vi "subSave_PatchParams_New.vi"(9 "Scaled output":cluster{"xo":i32, dbl, "data":dbl[][]}(graph)={"xo"=0, 5e-05, "data"=array2x40000[80000 elements]}, 10 "Patch quality":T1={"Ra (MΩ)"=236.79401827082728, "Rm (MΩ)"=5201.968657026799, "Cm (pF)"=4.323624616129607, "RC constant (msec)"=1.0238084463479926, "Steady state current (pA)"=9.611745724853648}, 11 "Base path":path=path "C:/Peng/Data/2014-05-13 neuron PZ066 DRH344/DRH344/fov2") -> ()   [LabVIEW 2015]
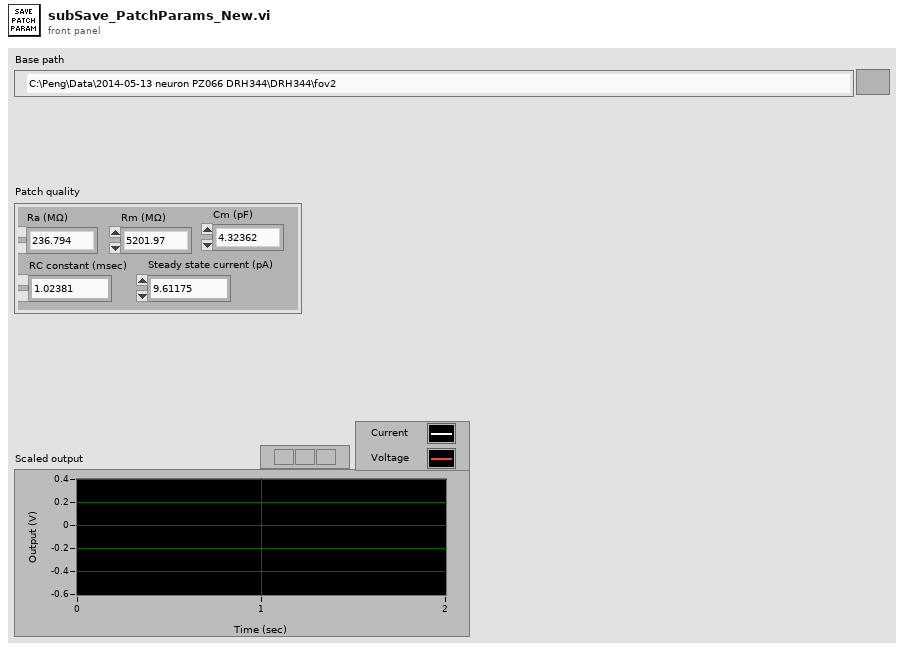
[diagram p1: front panel]
types:
  T1 = cluster{"Ra (MΩ)":dbl, "Rm (MΩ)":dbl, "Cm (pF)":dbl, "RC constant (msec)":dbl, "Steady state current (pA)":dbl}
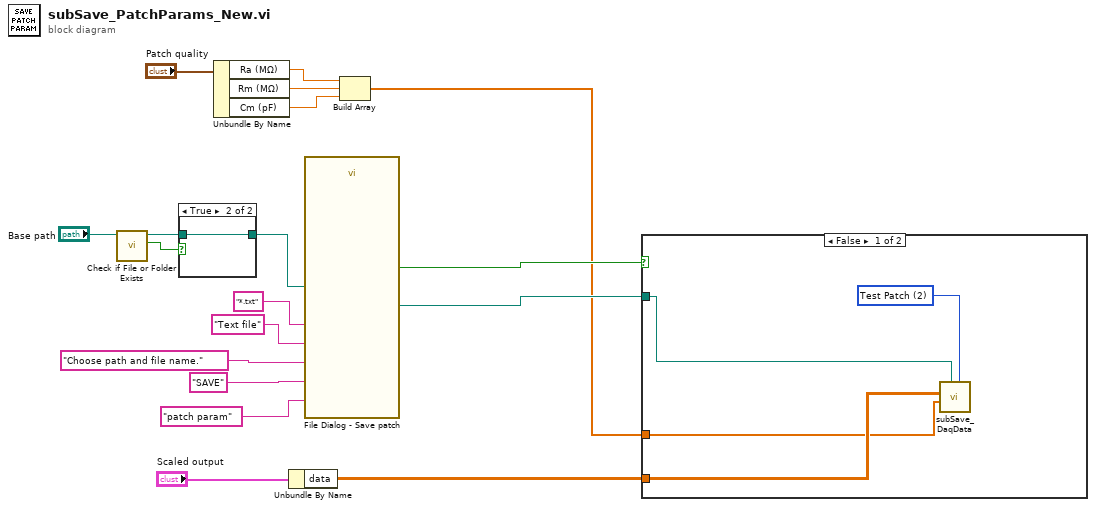
[diagram p0: block diagram]
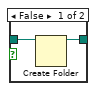
[diagram p3: hidden frame]
diagram:
  n1 = call <vilib>:"Check if File or Folder Exists.vi"("path"="Base path") -> ("file or folder exists?"=w11:bool, "dup path"=w12:path)  [unwired: 8 in, 1 out]
  n2 = case shown="True" w11 {
    tunnel: w12 -> [w20 w21]
    tunnel: [w19 w21] -> w9
    frame False {
      n3 = Create Folder(path (use dialog)=w20) -> (created path=w19:path)  [unwired: 2 in, 2 out]
    }
    frame True {
    }
  }
  n4 = Unbundle By Name("Patch quality") -> ("Ra (MΩ)"=w4:dbl, "Rm (MΩ)"=w3:dbl, "Cm (pF)"=w2:dbl)
  n5 = Unbundle By Name("Scaled output") -> ("data"=w6:dbl[][])
  n6 = call "File Dialog - Save patch"("start path"=w9, "prompt"="Choose path and file name.", "button label"="SAVE", "default name"="patch param" ("button label"), "pattern (all files)"="*.txt" ("default name"), "pattern label"="Text file" ("default name")) -> ("selected path"=w13:path, "cancelled"=w8:bool)  [unwired: 6 in, 2 out]
  n7 = Build Array(w4, w3, w2) -> (w1:dbl[])
  n8 = case shown="False" w8 {
    tunnel: w13 -> [w22 _]
    tunnel: w6 -> [w25 _]
    tunnel: w1 -> [w23 _]
    frame False {
      w24 = u16 2 items=["Complete waveforms", "Analog In only", "Test Patch"] ("Waveform type")
      n9 = call "subSave_DaqData.vi"("Waveform type (complete)"=w24, "path"=w22, "Test Patch array"=w23, "AI waveform"=w25) -> ()  [unwired: 7 in, 1 out]
    }
    frame True {
    }
  }
